vi "Load State Machine.vi"   [LabVIEW 2013]
uses:
  typedefs/fg_typedef.ctl
  typedefs/State Machine/singleUseSubstate.ctl
  <vilib>/Rock Robotics/WPI/Solenoid/WPI_SolenoidValue.ctl
  typedefs/DevRef Type.ctl
  typedefs/State Machine/subStates.ctl
  <vilib>/Rock Robotics/WPI/Solenoid/WPI_SolenoidGetEnum.vi
panel:
  # "A State Machine to Handle Loading for Either High or Low Goal Shots"
types:
  T1 = typedef "fg_typedef.ctl" = enum16{"Get", "Set"}
  T2 = typedef "DevRef Type.ctl" = enum16{"Shooter Solenoid", "Latch Solenoid", "Right Up Sensor", "Right Down Sensor", "Hold Sensor", "2 Ball Switch", "Arm Encoder"}
  T3 = typedef "WPI_SolenoidValue.ctl" = enum16{"Off", "On", "Forward", "Reverse"}
  T4 = typedef "singleUseSubstate.ctl" = enum16{"null", "wait", "shift high", "shift low", "extend shooter", "retract shooter", "latch", "unlatch", "end"}
  T5 = typedef "subStates.ctl" = enum16{"null", "wait", "driver control", "auto", "manual override", "hold position", "rotate", "pickup", "pass", "load", "goto shoot", "shoot high goal", "shoot low goal", "cancel arm", "cancel shooter", "end", "test"}
  T6 = typedef "WPI_SolenoidDevRef.ctl" = cluster{"DevStatus":errorcluster, "Solenoid Module":T7, "Forward Solenoid Channel":T8, "Reverse Solenoid Channel":T8}
  T7 = typedef "FPGA_TypedefSolenoidModule.ctl" = enum16{"Solenoid Module 1", "Solenoid Module 2"}
  T8 = typedef "WPI_SolenoidChannel.ctl" = enum8{"Solenoid 1", "Solenoid 2", "Solenoid 3", "Solenoid 4", "Solenoid 5", "Solenoid 6", "Solenoid 7", "Solenoid 8", "Invalid"}
  T9 = typedef "WPI_DigitalInputDevRef.ctl" = cluster{"DevStatus":errorcluster, "DIO Channel":T10, "Digital Module":T11}
  T10 = typedef "FPGA_DIOChannel.ctl" = enum8{"DIO 1", "DIO 2", "DIO 3", "DIO 4", "DIO 5", "DIO 6", "DIO 7", "DIO 8", "DIO 9", "DIO 10", "DIO 11", "DIO 12", "DIO 13", "DIO 14", "Invalid"}
  T11 = typedef "FPGA_TypedefDigitalModule.ctl" = enum16{"Digital Module 1", "Digital Module 2"}
  T12 = typedef "WPI_EncoderDevRef.ctl" = cluster{"DevStatus":errorcluster, "EncoderIndex":T13, "CounterIndex":T14, "DistancePerCount":dbl, "Decoding Type":T15}
  T13 = typedef "FPGA_EncoderIdx.ctl" = enum8{"Enc 0", "Enc 1", "Enc 2", "Enc 3", "Invalid"}
  T14 = typedef "FPGA_CounterCtrSystemIndex.ctl" = enum8{"Ctr 0", "Ctr 1", "Ctr 2", "Ctr 3", "Ctr 4", "Ctr 5", "Ctr 6", "Ctr 7", "Invalid"}
  T15 = typedef "WPI_EncoderType.ctl" = enum16{"1x", "2x", "4x"}
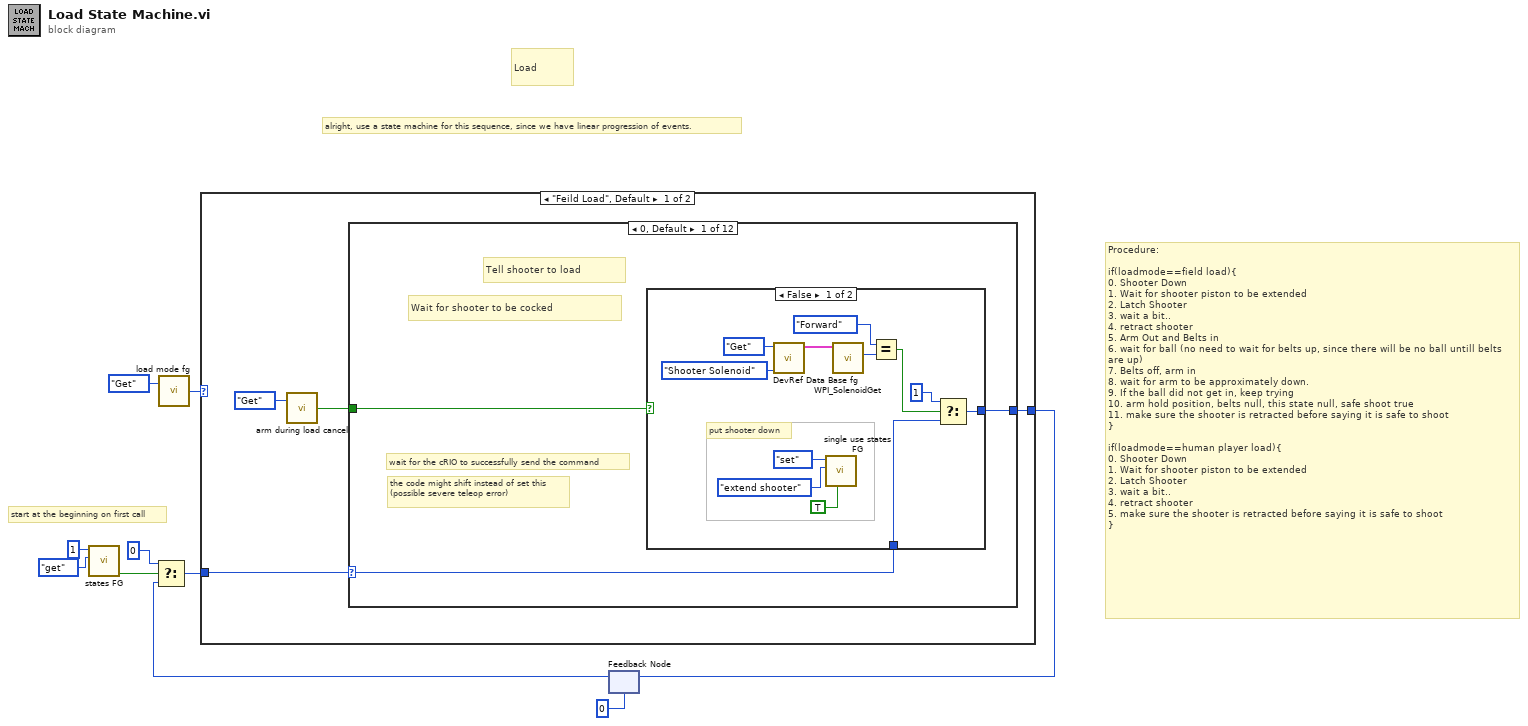
[diagram p0: block diagram]
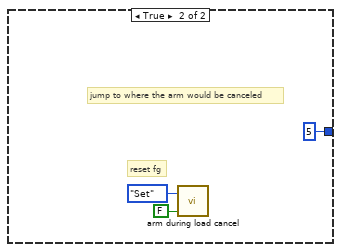
[diagram p2: hidden frame]
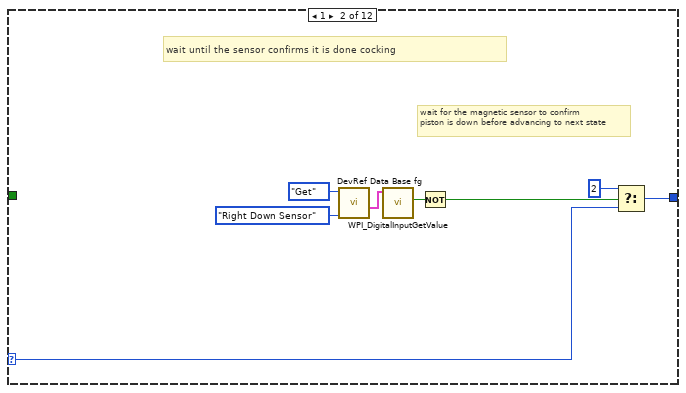
[diagram p3: hidden frame]
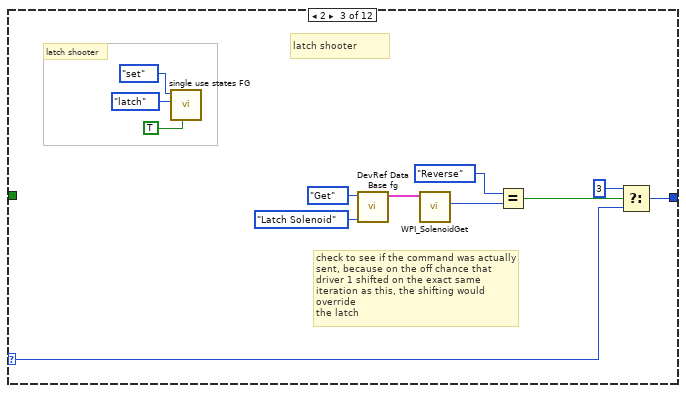
[diagram p4: hidden frame]
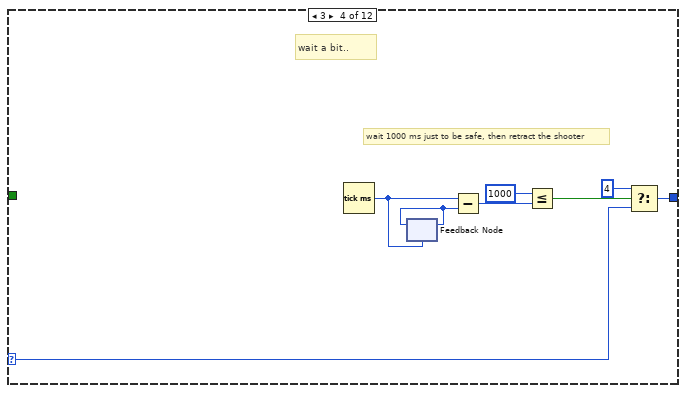
[diagram p5: hidden frame]
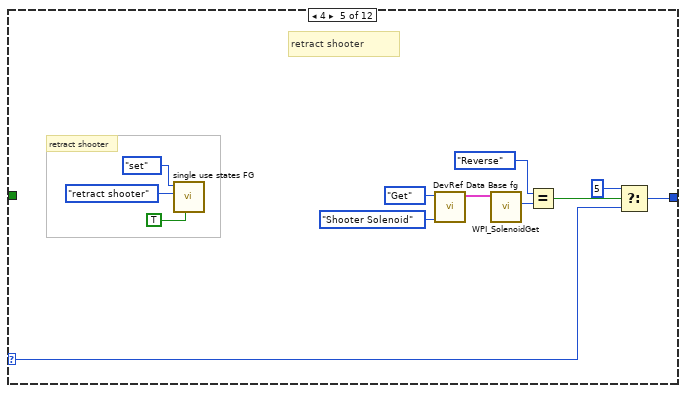
[diagram p6: hidden frame]
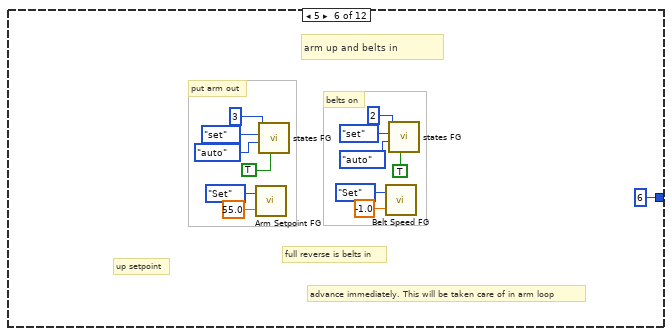
[diagram p7: hidden frame]
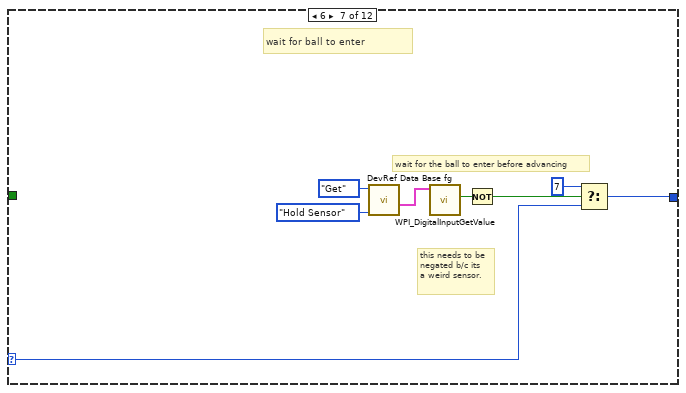
[diagram p8: hidden frame]
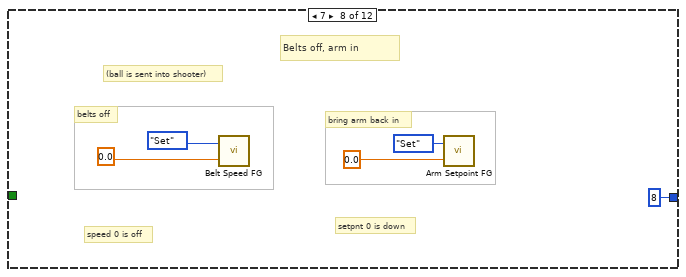
[diagram p9: hidden frame]
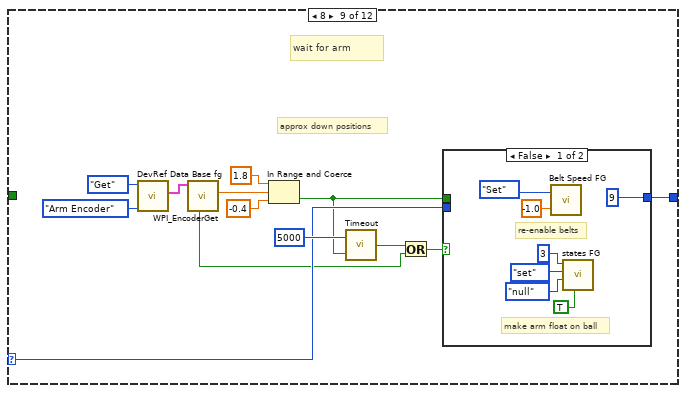
[diagram p10: hidden frame]
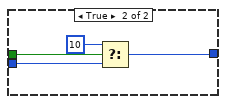
[diagram p11: hidden frame]
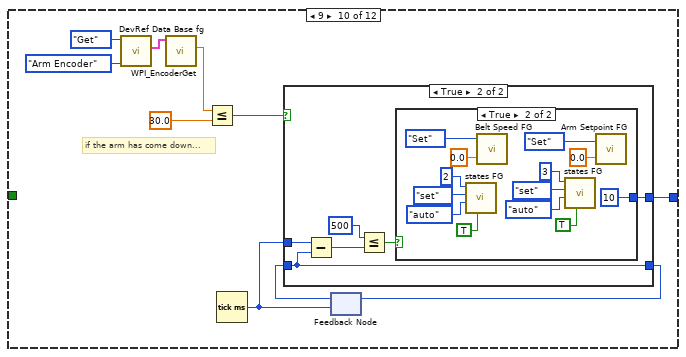
[diagram p12: hidden frame]
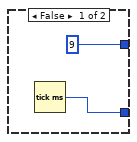
[diagram p13: hidden frame]
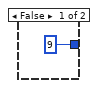
[diagram p14: hidden frame]
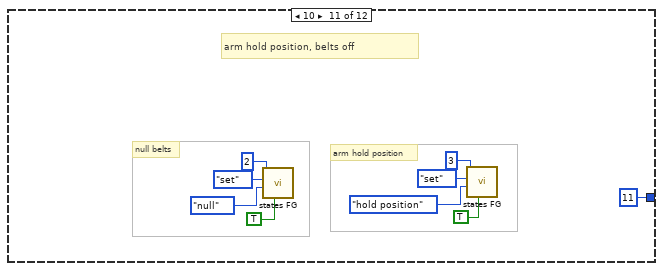
[diagram p15: hidden frame]
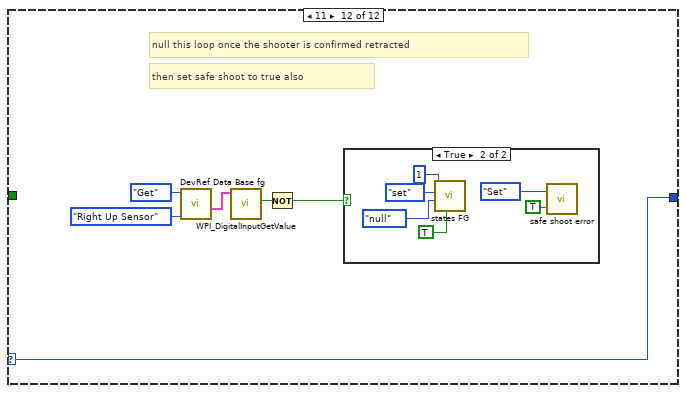
[diagram p16: hidden frame]
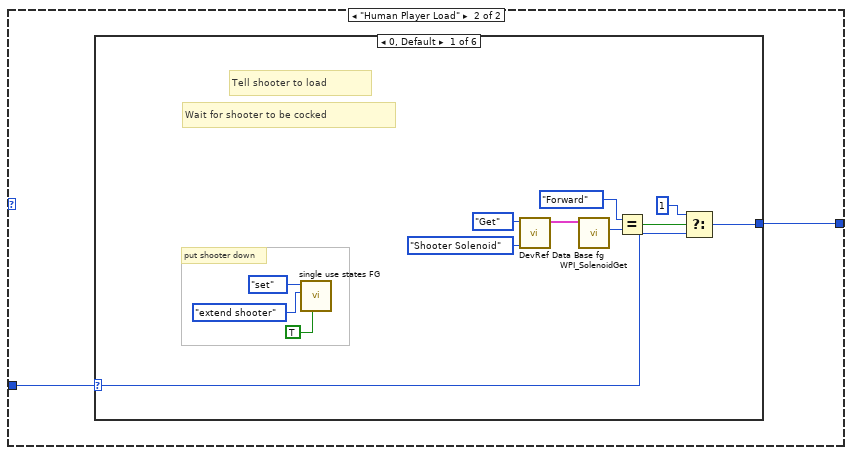
[diagram p18: hidden frame]
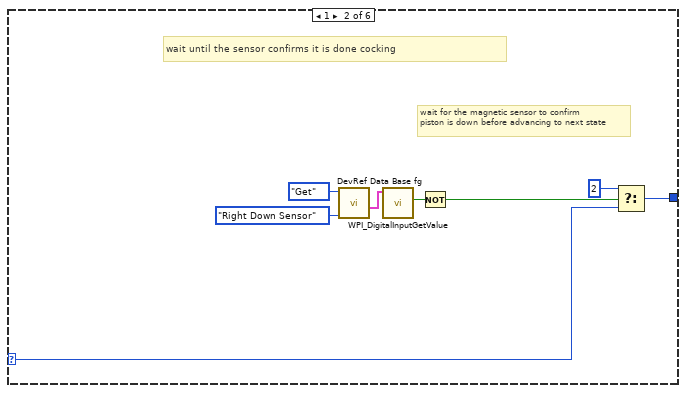
[diagram p19: hidden frame]
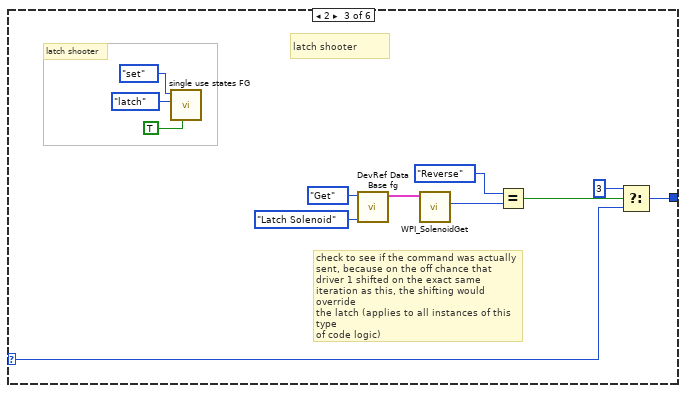
[diagram p20: hidden frame]
diagram:
  # "start at the beginning on first call"
  # "Load"
  # "Procedure: \n\nif(loadmode==field load){\n0. Shooter Down \n1. Wait for shooter piston to be extended\n2. Latch Shooter\n3. wait a bit..\n4. retract shooter\n5. Arm Out and Belts in\n6. wait for ball (no need to wait for belts up, since there will be no ball untill belts are up)\n7. Belts off, arm in\n8. wait for arm to be approximately down.\n9. If the ball did not get in, keep trying\n10. arm hold position, belts null, this state null, safe shoot true\n11. make sure the shooter is retracted before saying it is safe to shoot\n}\n\nif(loadmode==human player load){\n0. Shooter Down \n1. Wait for shooter piston to be extended\n2. Latch Shooter\n3. wait a bit..\n4. retract shooter\n5. make sure the shooter is retracted before saying it is safe to shoot\n}"
  # "alright, use a state machine for this sequence, since we have linear progression of events."
  n1 = call "states FG.vi"("menu (get)"=enum16{"set", "get"}."get", "Loop ID"=1) -> ("first call?"=w3:bool)  [unwired: 6 in, 3 out]
  n2 = call "load mode fg.vi"("Menu"=fg_typedef."Get") -> ("Load Mode"=w2:enum16{"Feild Load", "Human Player Load"})  [unwired: 1 in]
  n3 = feedback #1(u8 0) -> (w4:u8)
  n4 = Select(t=u8 0, s=w3, f=w4) -> (s? t:f=w6:u8)
  n5 = case shown="\"Feild Load\", Default" w2 {
    tunnel: [w14 w177] -> w9
    tunnel: w6 -> [w13 w176]
    frame "Feild Load", Default {
      n6 = call "arm during load cancel.vi"("Mode"=enum16{"Get", "Set", "Teleop Set"}."Get") -> ("Arm Canceled During Load"=w11:bool)  [unwired: 1 in]
      n7 = case shown="0, Default" w13 {
        selector: w13 -> [w16 w38 w48 w54 w69 _ w91 _ w103 _ _ w169]
        tunnel: [w17 w37 w49 w56 w68 u8 6 ("t") w90 u8 8 ("t") w104 w124 u8 11 ("t") w169] -> w14
        tunnel: w11 -> [w15 _ _ _ _ _ _ _ _ _ _ _]
        frame 0, Default {
          # "the code might shift instead of set this\n(possible severe teleop error)"
          # "Wait for shooter to be cocked"
          # "wait for the cRIO to successfully send the command"
          # "Tell shooter to load"
          n8 = case shown="False" w15 {
            tunnel: [w26 u8 5 ("t")] -> w17
            tunnel: w16 -> [w25 _]
            frame False {
              # "put shooter down"
              n9 = call "DevRef Data Base fg.vi"("DevRef to Get"=DevRef_Type."Shooter Solenoid", "Menu"=fg_typedef."Get") -> ("Selected Solenoid"=w24:T6)  [unwired: 2 in, 5 out]
              n10 = call "single use states FG.vi"("exit in"=TRUE, "substate"=singleUseSubstate."extend shooter", "menu (get)"=enum16{"set", "get"}."set") -> ()  [unwired: 5 in, 4 out]
              n11 = call-poly <vilib>:"WPI_SolenoidGet.vi"("SolenoidDevRef"=w24) -> ("Value"=w23:T3)  [unwired: 8 in, 2 out]
              n12 = Equal?(x=WPI_SolenoidValue."Forward", y=w23) -> (x = y?=w21:bool)
              n13 = Select(t=u8 1, s=w21, f=w25) -> (s? t:f=w26:u8)
            }
            frame True {
              # "reset fg"
              # "jump to where the arm would be canceled"
              n14 = call "arm during load cancel.vi"("Arm Canceled During Load?"=FALSE, "Mode"=enum16{"Get", "Set", "Teleop Set"}."Set") -> ()  [unwired: 1 out]
            }
          }
        }
        frame 1 {
          # "wait for the magnetic sensor to confirm \npiston is down before advancing to next state"
          # "wait until the sensor confirms it is done cocking"
          n15 = call "DevRef Data Base fg.vi"("DevRef to Get"=DevRef_Type."Right Down Sensor", "Menu"=fg_typedef."Get") -> ("Selected Sensor"=w39:T9)  [unwired: 2 in, 5 out]
          n16 = call <vilib>:"WPI_DigitalInputGetValue.vi"("DigitalInputDevRef"=w39) -> ("Value"=w40:bool)  [unwired: 8 in, 2 out]
          n17 = Not(x=w40) -> (.not. x?=w35:bool)
          n18 = Select(t=u8 2, s=w35, f=w38) -> (s? t:f=w37:u8)
        }
        frame 2 {
          # "latch shooter"
          # "check to see if the command was actually\nsent, because on the off chance that\ndriver 1 shifted on the exact same\niteration as this, the shifting would override\nthe latch"
          # "latch shooter"
          n19 = call "single use states FG.vi"("exit in"=TRUE, "substate"=singleUseSubstate."latch", "menu (get)"=enum16{"set", "get"}."set") -> ()  [unwired: 5 in, 4 out]
          n20 = call "DevRef Data Base fg.vi"("DevRef to Get"=DevRef_Type."Latch Solenoid", "Menu"=fg_typedef."Get") -> ("Selected Solenoid"=w47:T6)  [unwired: 2 in, 5 out]
          n21 = call-poly <vilib>:"WPI_SolenoidGet.vi"("SolenoidDevRef"=w47) -> ("Value"=w46:T3)  [unwired: 8 in, 2 out]
          n22 = Equal?(x=WPI_SolenoidValue."Reverse" ("Value"), y=w46) -> (x = y?=w44:bool)
          n23 = Select(t=u8 3, s=w44, f=w48) -> (s? t:f=w49:u8)
        }
        frame 3 {
          # "wait a bit.."
          # "wait 1000 ms just to be safe, then retract the shooter"
          n24 = Tick Count (ms)() -> (millisecond timer value=w58:u32)
          n25 = feedback #2(w58) -> (w59:u32)
          n26 = feedback-in #2(w59) -> ()
          n27 = Subtract(x=w58, y=w59) -> (x-y=w57:u32)
          n28 = Less Or Equal?(x=u32 1000, y=w57) -> (x <= y?=w55:bool)
          n29 = Select(t=u8 4, s=w55, f=w54) -> (s? t:f=w56:u8)
        }
        frame 4 {
          # "retract shooter"
          # "retract shooter"
          n30 = call "single use states FG.vi"("exit in"=TRUE, "substate"=singleUseSubstate."retract shooter", "menu (get)"=enum16{"set", "get"}."set") -> ()  [unwired: 5 in, 4 out]
          n31 = call "DevRef Data Base fg.vi"("DevRef to Get"=DevRef_Type."Shooter Solenoid", "Menu"=fg_typedef."Get") -> ("Selected Solenoid"=w67:T6)  [unwired: 2 in, 5 out]
          n32 = call-poly <vilib>:"WPI_SolenoidGet.vi"("SolenoidDevRef"=w67) -> ("Value"=w66:T3)  [unwired: 8 in, 2 out]
          n33 = Equal?(x=WPI_SolenoidValue."Reverse", y=w66) -> (x = y?=w64:bool)
          n34 = Select(t=u8 5, s=w64, f=w69) -> (s? t:f=w68:u8)
        }
        frame 5 {
          # "full reverse is belts in"
          # "belts on"
          # "up setpoint"
          # "arm up and belts in"
          # "advance immediately. This will be taken care of in arm loop"
          # "put arm out"
          n35 = call "Arm Setpoint FG.vi"("Setpoint In"=55.0, "Menu"=fg_typedef."Set") -> ()  [unwired: 1 out]
          n36 = call "states FG.vi"("exit in"=TRUE, "subState in"=subStates."auto", "menu (get)"=enum16{"set", "get"}."set", "Loop ID"=3) -> ()  [unwired: 4 in, 4 out]
          n37 = call "Belt Speed FG.vi"("Speed In"=-1.0 ("Setpoint In"), "Menu"=fg_typedef."Set") -> ()  [unwired: 1 out]
          n38 = call "states FG.vi"("exit in"=TRUE, "subState in"=subStates."auto", "menu (get)"=enum16{"set", "get"}."set", "Loop ID"=2) -> ()  [unwired: 4 in, 4 out]
        }
        frame 6 {
          # "this needs to be\nnegated b/c its\na weird sensor."
          # "wait for the ball to enter before advancing"
          # "wait for ball to enter"
          n39 = call "DevRef Data Base fg.vi"("DevRef to Get"=DevRef_Type."Hold Sensor", "Menu"=fg_typedef."Get") -> ("Selected Sensor"=w89:T9)  [unwired: 2 in, 5 out]
          n40 = call <vilib>:"WPI_DigitalInputGetValue.vi"("DigitalInputDevRef"=w89) -> ("Value"=w93:bool)  [unwired: 8 in, 2 out]
          n41 = Not(x=w93) -> (.not. x?=w92:bool)
          n42 = Select(t=u8 7, s=w92, f=w91) -> (s? t:f=w90:u8)
        }
        frame 7 {
          # "bring arm back in"
          # "setpnt 0 is down"
          # "speed 0 is off"
          # "Belts off, arm in"
          # "(ball is sent into shooter)"
          # "belts off"
          n43 = call "Belt Speed FG.vi"("Speed In"=0.0 ("Setpoint In"), "Menu"=fg_typedef."Set") -> ()  [unwired: 1 out]
          n44 = call "Arm Setpoint FG.vi"("Setpoint In"=0.0, "Menu"=fg_typedef."Set") -> ()  [unwired: 1 out]
        }
        frame 8 {
          # "approx down positions"
          # "wait for arm"
          n45 = call "DevRef Data Base fg.vi"("DevRef to Get"=DevRef_Type."Arm Encoder", "Menu"=fg_typedef."Get") -> ("Selected Encoder"=w111:T12)  [unwired: 2 in, 5 out]
          n46 = call <vilib>:"WPI_EncoderGet.vi"("EncoderDevRef"=w111) -> ("Distance"=w110:dbl, "Stopped"=w99:bool)  [unwired: 5 in, 4 out]
          n47 = In Range and Coerce(upper limit=1.8, x=w110, lower limit=-0.4) -> (In Range?=w102:bool)  [unwired: 1 out]
          n48 = call "Timeout.vi"("Done with Task?"=w102, "Timeout (ms)"=u32 5000) -> ("Timed Out?"=w100:bool)  [unwired: 1 in]
          n49 = Or(x=w100, y=w99) -> (x .or. y?=w101:bool)
          n50 = case shown="False" w101 {
            tunnel: w103 -> [_ w122]
            tunnel: [u8 9 ("t") w121] -> w104
            tunnel: w102 -> [_ w119]
            frame False {
              # "re-enable belts"
              # "make arm float on ball"
              n51 = call "Belt Speed FG.vi"("Speed In"=-1.0, "Menu"=fg_typedef."Set") -> ()  [unwired: 1 out]
              n52 = call "states FG.vi"("exit in"=TRUE, "subState in"=subStates."null", "menu (get)"=enum16{"set", "get"}."set", "Loop ID"=3) -> ()  [unwired: 4 in, 4 out]
            }
            frame True {
              n53 = Select(t=u8 10, s=w119, f=w122) -> (s? t:f=w121:u8)
            }
          }
        }
        frame 9 {
          # "if the arm has come down..."
          n54 = call "DevRef Data Base fg.vi"("DevRef to Get"=DevRef_Type."Arm Encoder", "Menu"=fg_typedef."Get") -> ("Selected Encoder"=w128:T12)  [unwired: 2 in, 5 out]
          n55 = call <vilib>:"WPI_EncoderGet.vi"("EncoderDevRef"=w128) -> ("Distance"=w132:dbl)  [unwired: 5 in, 5 out]
          n56 = Less Or Equal?(x=w132, y=30.0) -> (x <= y?=w123:bool)
          n57 = Tick Count (ms)() -> (millisecond timer value=w126:u32)
          n58 = feedback #3(w126) -> (w127:u32)
          n59 = case shown="True" w123 {
            tunnel: [w134 w140] -> w125
            tunnel: w127 -> [_ w140]
            tunnel: w126 -> [_ w139]
            tunnel: [u8 9 w135] -> w124
            frame False {
              n60 = Tick Count (ms)() -> (millisecond timer value=w134:u32)
            }
            frame True {
              n61 = Subtract(x=w139, y=w140) -> (x-y=w138:u32)
              n62 = Less Or Equal?(x=u32 500, y=w138) -> (x <= y?=w136:bool)
              n63 = case shown="True" w136 {
                tunnel: [u8 9 u8 10] -> w135
                frame False {
                }
                frame True {
                  n64 = call "states FG.vi"("exit in"=TRUE, "subState in"=subStates."auto", "menu (get)"=enum16{"set", "get"}."set", "Loop ID"=2) -> ()  [unwired: 4 in, 4 out]
                  n65 = call "Belt Speed FG.vi"("Speed In"=0.0, "Menu"=fg_typedef."Set") -> ()  [unwired: 1 out]
                  n66 = call "states FG.vi"("exit in"=TRUE, "subState in"=subStates."auto", "menu (get)"=enum16{"set", "get"}."set", "Loop ID"=3) -> ()  [unwired: 4 in, 4 out]
                  n67 = call "Arm Setpoint FG.vi"("Setpoint In"=0.0, "Menu"=fg_typedef."Set") -> ()  [unwired: 1 out]
                }
              }
            }
          }
          n68 = feedback-in #3(w125) -> ()
        }
        frame 10 {
          # "null belts"
          # "arm hold position, belts off"
          # "arm hold position"
          n69 = call "states FG.vi"("exit in"=TRUE, "subState in"=subStates."null", "menu (get)"=enum16{"set", "get"}."set", "Loop ID"=2) -> ()  [unwired: 4 in, 4 out]
          n70 = call "states FG.vi"("exit in"=TRUE, "subState in"=subStates."hold position", "menu (get)"=enum16{"set", "get"}."set", "Loop ID"=3) -> ()  [unwired: 4 in, 4 out]
        }
        frame 11 {
          # "then set safe shoot to true also"
          # "null this loop once the shooter is confirmed retracted"
          n71 = call "DevRef Data Base fg.vi"("DevRef to Get"=DevRef_Type."Right Up Sensor", "Menu"=fg_typedef."Get") -> ("Selected Sensor"=w168:T9)  [unwired: 2 in, 5 out]
          n72 = call <vilib>:"WPI_DigitalInputGetValue.vi"("DigitalInputDevRef"=w168) -> ("Value"=w167:bool)  [unwired: 8 in, 2 out]
          n73 = Not(x=w167) -> (.not. x?=w166:bool)
          n74 = case shown="True" w166 {
            frame False {
            }
            frame True {
              n75 = call "states FG.vi"("exit in"=TRUE, "subState in"=subStates."null", "menu (get)"=enum16{"set", "get"}."set", "Loop ID"=1) -> ()  [unwired: 4 in, 4 out]
              n76 = call "safe shoot error.vi"("Can Shoot Safely?"=TRUE, "Menu"=fg_typedef."Set") -> ()  [unwired: 1 out]
            }
          }
        }
      }
    }
    frame "Human Player Load" {
      n77 = case shown="0, Default" w176 {
        selector: w176 -> [w188 w195 w205 w211 w226 w237]
        tunnel: [w189 w194 w206 w213 w225 w237] -> w177
        frame 0, Default {
          # "put shooter down"
          # "Wait for shooter to be cocked"
          # "Tell shooter to load"
          n78 = call "single use states FG.vi"("exit in"=TRUE, "substate"=singleUseSubstate."extend shooter", "menu (get)"=enum16{"set", "get"}."set") -> ()  [unwired: 5 in, 4 out]
          n79 = call "DevRef Data Base fg.vi"("DevRef to Get"=DevRef_Type."Shooter Solenoid", "Menu"=fg_typedef."Get") -> ("Selected Solenoid"=w184:T6)  [unwired: 2 in, 5 out]
          n80 = call-poly <vilib>:"WPI_SolenoidGet.vi"("SolenoidDevRef"=w184) -> ("Value"=w183:T3)  [unwired: 8 in, 2 out]
          n81 = Equal?(x=WPI_SolenoidValue."Forward", y=w183) -> (x = y?=w181:bool)
          n82 = Select(t=u8 1, s=w181, f=w188) -> (s? t:f=w189:u8)
        }
        frame 1 {
          # "wait for the magnetic sensor to confirm \npiston is down before advancing to next state"
          # "wait until the sensor confirms it is done cocking"
          n83 = call "DevRef Data Base fg.vi"("DevRef to Get"=DevRef_Type."Right Down Sensor", "Menu"=fg_typedef."Get") -> ("Selected Sensor"=w196:T9)  [unwired: 2 in, 5 out]
          n84 = call <vilib>:"WPI_DigitalInputGetValue.vi"("DigitalInputDevRef"=w196) -> ("Value"=w197:bool)  [unwired: 8 in, 2 out]
          n85 = Not(x=w197) -> (.not. x?=w192:bool)
          n86 = Select(t=u8 2, s=w192, f=w195) -> (s? t:f=w194:u8)
        }
        frame 2 {
          # "latch shooter"
          # "check to see if the command was actually\nsent, because on the off chance that\ndriver 1 shifted on the exact same\niteration as this, the shifting would override\nthe latch (applies to all instances of this type\nof code logic)"
          # "latch shooter"
          n87 = call "single use states FG.vi"("exit in"=TRUE, "substate"=singleUseSubstate."latch", "menu (get)"=enum16{"set", "get"}."set") -> ()  [unwired: 5 in, 4 out]
          n88 = call "DevRef Data Base fg.vi"("DevRef to Get"=DevRef_Type."Latch Solenoid", "Menu"=fg_typedef."Get") -> ("Selected Solenoid"=w204:T6)  [unwired: 2 in, 5 out]
          n89 = call-poly <vilib>:"WPI_SolenoidGet.vi"("SolenoidDevRef"=w204) -> ("Value"=w203:T3)  [unwired: 8 in, 2 out]
          n90 = Equal?(x=WPI_SolenoidValue."Reverse" ("Value"), y=w203) -> (x = y?=w201:bool)
          n91 = Select(t=u8 3, s=w201, f=w205) -> (s? t:f=w206:u8)
        }
        frame 3 {
          # "wait a bit.."
          # "wait 1000 ms just to be safe, then retract the shooter"
          n92 = Tick Count (ms)() -> (millisecond timer value=w215:u32)
          n93 = feedback #4(w215) -> (w216:u32)
          n94 = feedback-in #4(w216) -> ()
          n95 = Subtract(x=w215, y=w216) -> (x-y=w214:u32)
          n96 = Less Or Equal?(x=u32 1000, y=w214) -> (x <= y?=w212:bool)
          n97 = Select(t=u8 4, s=w212, f=w211) -> (s? t:f=w213:u8)
        }
        frame 4 {
          # "retract shooter"
          # "retract shooter"
          n98 = call "single use states FG.vi"("exit in"=TRUE, "substate"=singleUseSubstate."retract shooter", "menu (get)"=enum16{"set", "get"}."set") -> ()  [unwired: 5 in, 4 out]
          n99 = call "DevRef Data Base fg.vi"("DevRef to Get"=DevRef_Type."Shooter Solenoid", "Menu"=fg_typedef."Get") -> ("Selected Solenoid"=w224:T6)  [unwired: 2 in, 5 out]
          n100 = call-poly <vilib>:"WPI_SolenoidGet.vi"("SolenoidDevRef"=w224) -> ("Value"=w223:T3)  [unwired: 8 in, 2 out]
          n101 = Equal?(x=WPI_SolenoidValue."Reverse", y=w223) -> (x = y?=w221:bool)
          n102 = Select(t=u8 5, s=w221, f=w226) -> (s? t:f=w225:u8)
        }
        frame 5 {
          # "set this false here because it is never\nsupposed to be hit during this type of load\nsince the arm is not used"
          # "then set safe shoot to true also"
          # "null this loop once the shooter is confirmed retracted"
          n103 = call "arm during load cancel.vi"("Arm Canceled During Load?"=FALSE, "Mode"=enum16{"Get", "Set", "Teleop Set"}."Set") -> ()  [unwired: 1 out]
          n104 = call "DevRef Data Base fg.vi"("DevRef to Get"=DevRef_Type."Right Up Sensor", "Menu"=fg_typedef."Get") -> ("Selected Sensor"=w236:T9)  [unwired: 2 in, 5 out]
          n105 = call <vilib>:"WPI_DigitalInputGetValue.vi"("DigitalInputDevRef"=w236) -> ("Value"=w235:bool)  [unwired: 8 in, 2 out]
          n106 = Not(x=w235) -> (.not. x?=w234:bool)
          n107 = case shown="True" w234 {
            frame False {
            }
            frame True {
              n108 = call "states FG.vi"("exit in"=TRUE, "subState in"=subStates."null", "menu (get)"=enum16{"set", "get"}."set", "Loop ID"=1) -> ()  [unwired: 4 in, 4 out]
              n109 = call "safe shoot error.vi"("Can Shoot Safely?"=TRUE, "Menu"=fg_typedef."Set") -> ()  [unwired: 1 out]
            }
          }
        }
      }
    }
  }
  n110 = feedback-in #1(w9) -> ()
